vi "HandleErrors.vi"() -> ()   [LabVIEW 2019]
uses:
  Error handler_class/Error handler.lvclass
panel:
  in  "Testing":bool=TRUE
  in  "Show Error Window on Error":bool=TRUE
  out "Error Indication":bool
  in  "error message (\"\")":string
  in  "code":i32
  in  "Status":bool=TRUE
  in  "UnknownError":bool
  in  "KnownError":bool
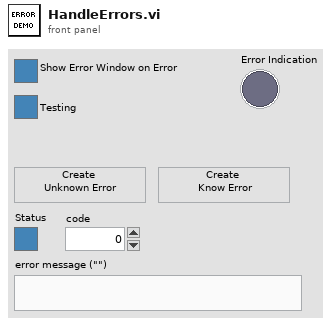
[diagram p1: front panel]
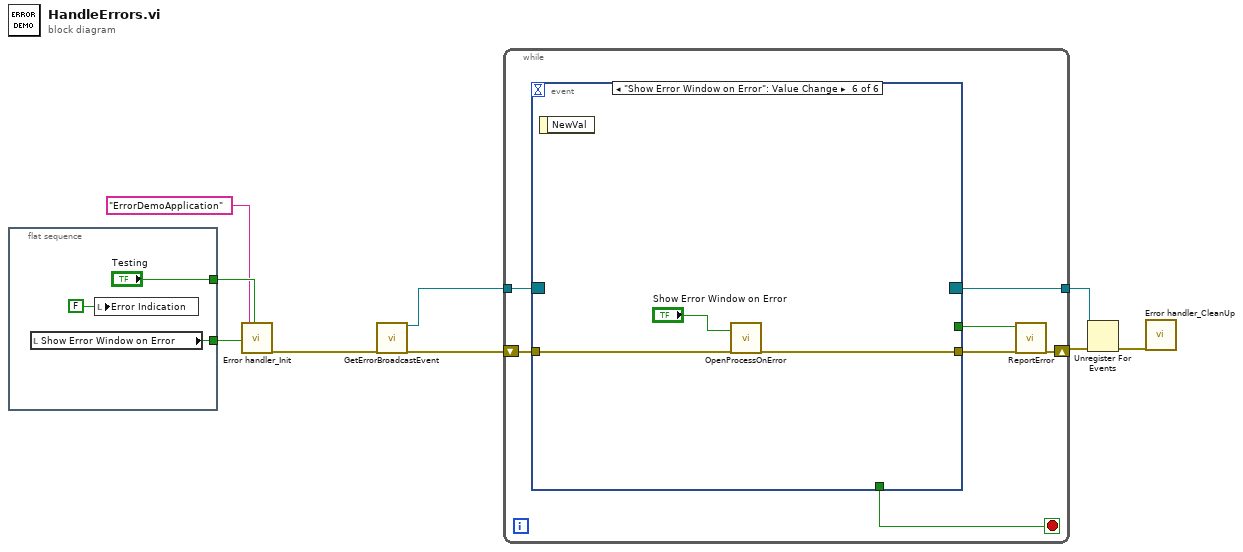
[diagram p0: block diagram]
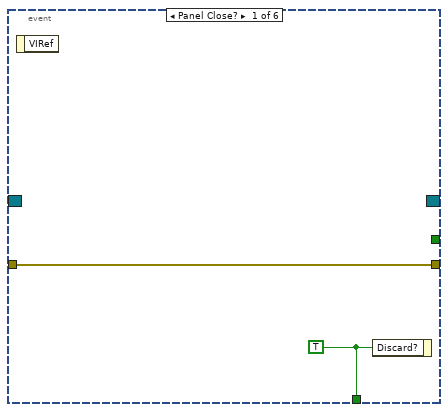
[diagram p2: hidden frame]
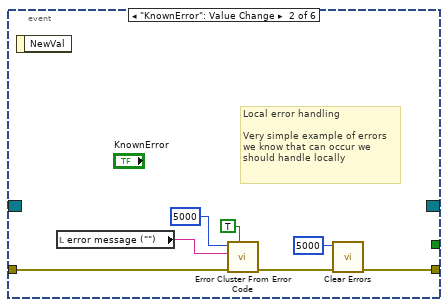
[diagram p3: hidden frame]
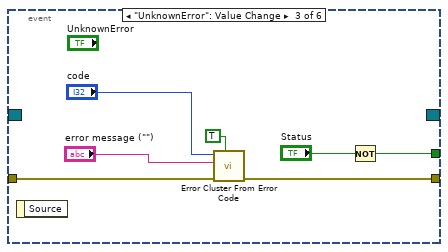
[diagram p4: hidden frame]
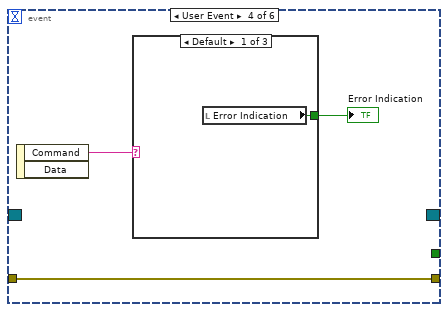
[diagram p5: hidden frame]
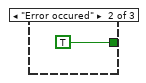
[diagram p6: hidden frame]
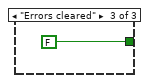
[diagram p7: hidden frame]
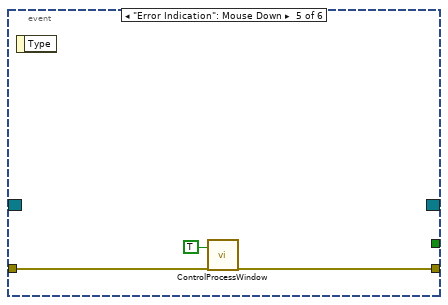
[diagram p8: hidden frame]
diagram:
  n1 = flat-sequence {
    tunnel: [w12] -> w4
    tunnel: ["Testing"] -> w2
    frame #0 {
      n2 = local read "Show Error Window on Error"() -> (w12:bool)
      n3 = local write "Error Indication"(FALSE ("Error hänt")) -> ()
    }
  }
  n4 = call "Error handler_Init.vi"("LoadFPOnError"=w4, "Name"="ErrorDemoApplication", "Testing"=w2) -> ("Error Out"=w8:errorcluster)  [unwired: 15 in, 1 out]
  n5 = call "GetErrorBroadcastEvent.vi"("Error In"=w8) -> ("ErrorBroadcastEvent"=w3:refnum<event-registration>, "Error Out"=w7:errorcluster)  [unwired: 17 in]
  n6 = while {
    shift-right: [w16] -> w9
    shift-left: w7 -> [w18]
    tunnel: [w14] -> w5
    tunnel: w3 -> [w13]
    stop <- w19 stop-if-true
    n7 = event shown="[5] \"Show Error Window on Error\": Value Change" {
      selector: w13 -> [_ _ _ _ _ _]
      dyn-events: [_ _ _ _ _ _] -> w14
      timeout: _ -> [_ _ _ _ _ _]
      tunnel: [w21 _ _ _ _ _] -> w19
      tunnel: w18 -> [w20 w25 w33 w38 w44 w47]
      tunnel: [w20 w28 w32 w38 w43 w46] -> w17
      tunnel: [_ _ w30 _ _ _] -> w15
      event Panel Close? {
        w21 = TRUE ("Discard?")
        n8 = event-data() -> ()  [unwired: 1 in, 1 out]
        n9 = event-data("Discard?"=w21) -> ()  [unwired: 1 in, 1 out]
      }
      event "KnownError": Value Change {
        # "Local error handling\n\nVery simple example of errors we know that can occur we should handle locally"
        n10 = event-data() -> ()  [unwired: 1 in, 1 out]
        n11 = local read "error message (\"\")"() -> (w23:string)
        n12 = call <vilib>:"Error Cluster From Error Code.vi"("show call chain? (False)"=TRUE, "error in (no error)"=w25, "error message (\"\")"=w23, "error code (0)"=5000 ("code")) -> ("error out"=w26:errorcluster)  [unwired: 5 in]
        n13 = call <vilib>:"Clear Errors.vi"("error in (no error)"=w26, "specific error code to clear (0: all)"=5000) -> ("error out"=w28:errorcluster)  [unwired: 4 in, 1 out]
      }
      event "UnknownError": Value Change {
        n14 = event-data() -> ()  [unwired: 1 in, 1 out]
        n15 = call <vilib>:"Error Cluster From Error Code.vi"("show call chain? (False)"=TRUE, "error in (no error)"=w33, "error message (\"\")"="error message (\"\")", "error code (0)"="code") -> ("error out"=w32:errorcluster)  [unwired: 5 in]
        n16 = Not(x="Status") -> (.not. x?=w30:bool)
      }
      event User Event {
        n17 = event-data() -> ("Command"=w37:string)  [unwired: 1 in, 1 out]
        n18 = case shown="Default" w37 {
          tunnel: [w39 TRUE ("Status") FALSE ("Status")] -> w36
          frame Default {
            n19 = local read "Error Indication"() -> (w39:bool)
          }
          frame "Error occured" {
          }
          frame "Errors cleared" {
          }
        }
        "Error Indication" <- w36
      }
      event "Error Indication": Mouse Down {
        n20 = event-data() -> ()  [unwired: 1 in, 1 out]
        n21 = call "ControlProcessWindow.vi"("ShowProcessWindow"=TRUE, "Error In"=w44) -> ("Error Out"=w43:errorcluster)  [unwired: 17 in]
      }
      event "Show Error Window on Error": Value Change {
        n22 = event-data() -> ()  [unwired: 1 in, 1 out]
        n23 = call "OpenProcessOnError.vi"("Open?"="Show Error Window on Error", "Error In"=w47) -> ("Error Out"=w46:errorcluster)  [unwired: 17 in]
      }
    }
    n24 = call "ReportError.vi"("Convert to warning"=w15, "Error In"=w17) -> ("Error Out"=w16:errorcluster)  [unwired: 17 in]
  }
  n25 = Unregister For Events(event registration refnum=w5, error in=w9) -> (error out=w6:errorcluster)
  n26 = call "Error handler_CleanUp.vi"("Error In"=w6) -> ()  [unwired: 18 in, 1 out]
